vi "Check Time.vi"(11 "Logging Configuration":T1={"Log File Base Path"=path "", "TDMS File Reference"=refnum, "Reset"=FALSE, "Wait"=0.0, "Start Time"=0.0, "Update Rate"=1, "Channel Names"=[], "System Preset"=variant} {"Update Rate" min=1 max=10 step=1}) -> (1 "Time has Elapsed":bool, 2 "Elapsed Time (s)":dbl, 3 "Logging Configuration out":T1={"Log File Base Path"=path "", "TDMS File Reference"=refnum, "Reset"=FALSE, "Wait"=0.0, "Start Time"=0.0, "Update Rate"=1, "Channel Names"=[], "System Preset"=variant} {"Update Rate" min=1 max=10 step=1})   [LabVIEW 2020, in "SAVE.lvlib"]
uses:
  SAVE.lvlib
  Save Configuration.ctl
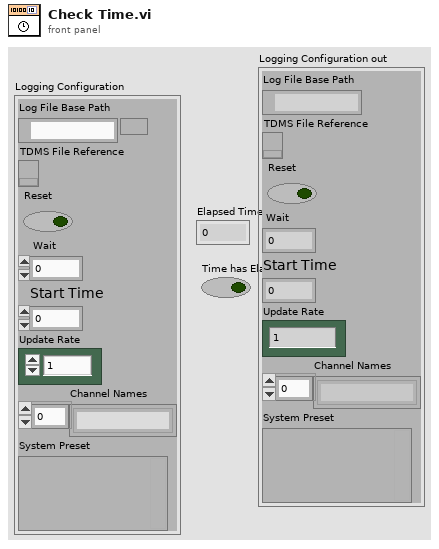
[diagram p1: front panel]
types:
  T1 = typedef "SAVE.lvlib/Save Configuration.ctl" = cluster{"Log File Base Path":path, "TDMS File Reference":refnum<k34>, "Reset":bool, "Wait":dbl, "Start Time":dbl, "Update Rate":u16, "Channel Names":string[], "System Preset":variant}
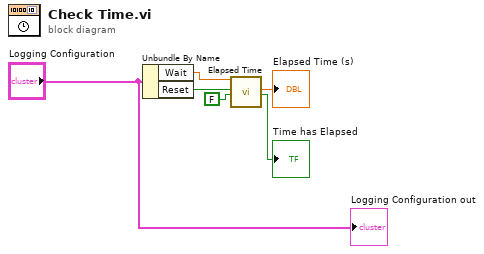
[diagram p0: block diagram]
diagram:
  n1 = Unbundle By Name("Logging Configuration") -> ("Wait"=w6:dbl, "Reset"=w4:bool)
  n2 = call "Elapsed Time"("Time Target (s)"=w6, "Reset"=w4, "Auto Reset"=FALSE) -> ("Elapsed Time (s)"=→"Elapsed Time (s)":dbl, "Time has Elapsed"=→"Time has Elapsed":bool)  [unwired: 9 in, 6 out]
  "Logging Configuration out" <- "Logging Configuration"
